vi "ServoController_check.vi"(7 "Servo Position Old (U16)":u16[][](array[numeric]), 8 "Error In":errorcluster, 11 "Servo Position In (U16)":u16[][](array[numeric])) -> (0 "Error Out":errorcluster, 3 "Servo Position Out (U16)":u16[][](array[numeric]))   [LabVIEW 2013]
uses:
  My Computer/Controls/Fin Status.ctl
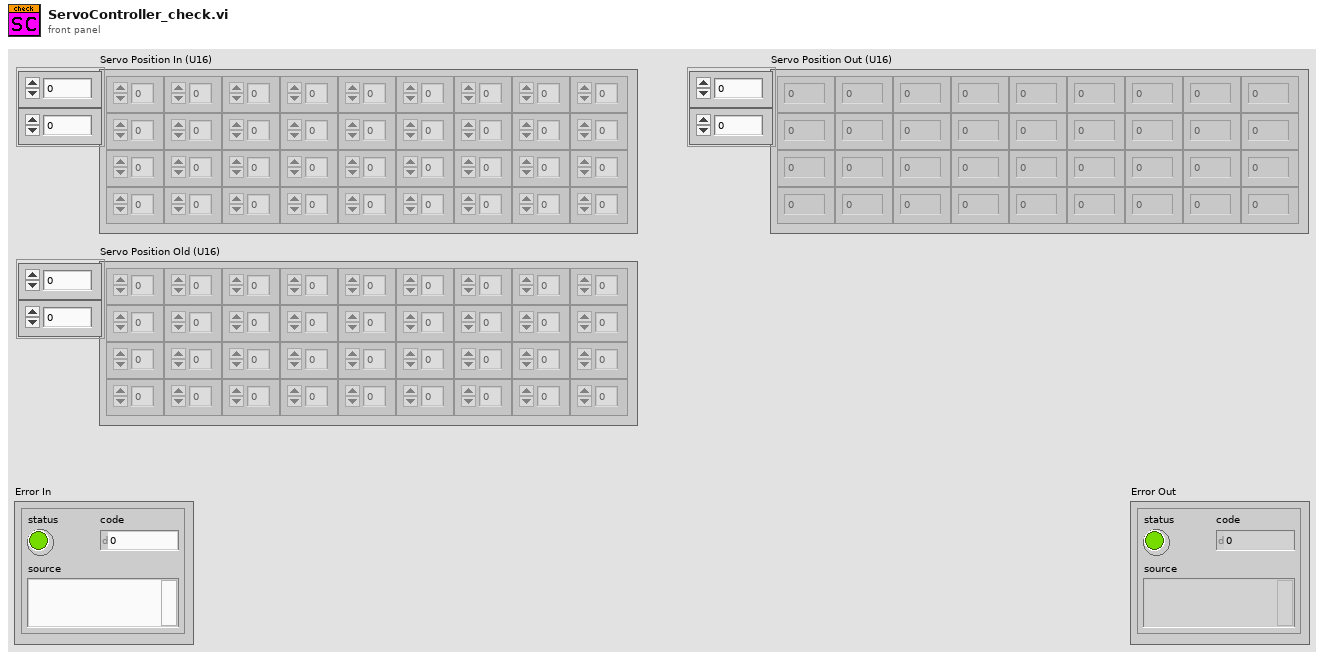
[diagram p1: front panel]
types:
  T1 = typedef "Fin Status.ctl" = u32[]
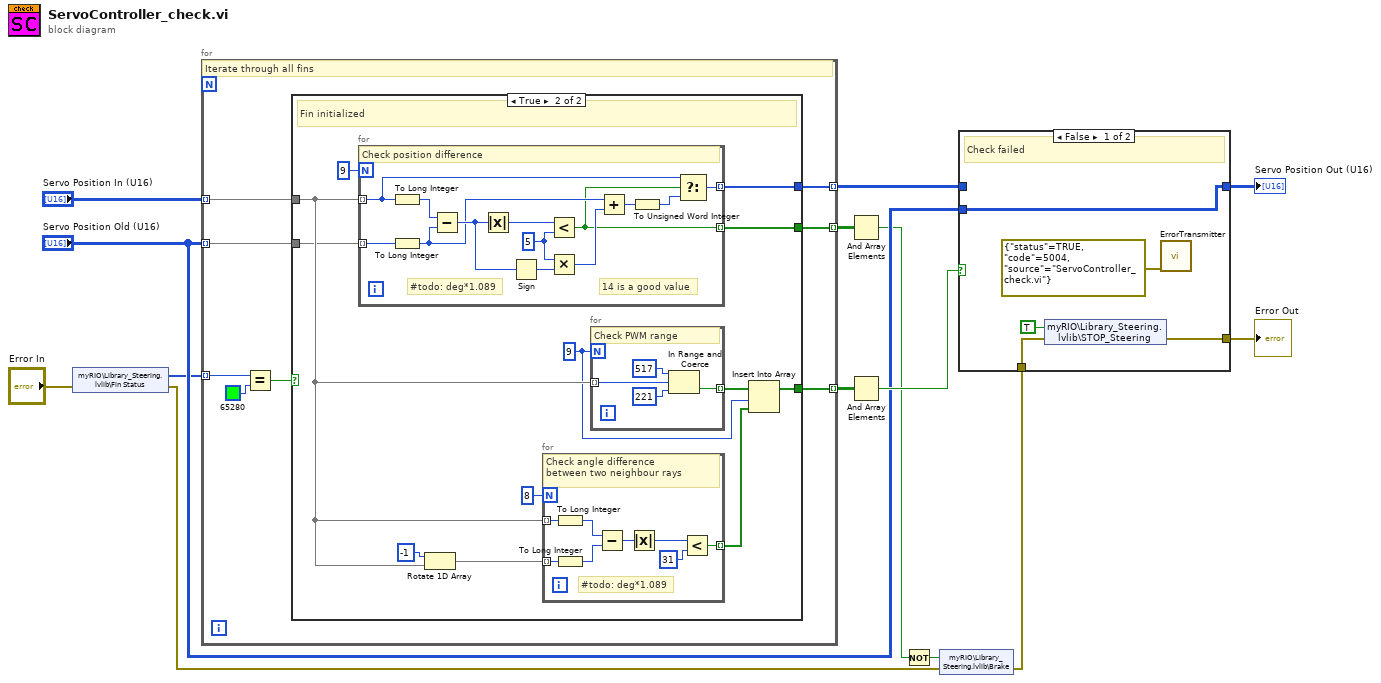
[diagram p0: block diagram]
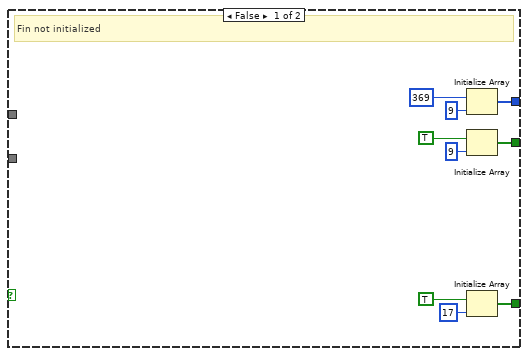
[diagram p3: hidden frame]
diagram:
  n1 = shared-variable "myRIO\\Library_Steering.lvlib\\Fin Status"(error in="Error In") -> (w8:T1, error out=w4:errorcluster)
  n2 = for {
    tunnel: [w22] -> w10 mode=indexing
    tunnel: "Servo Position In (U16)" -> [w21] mode=indexing
    tunnel: "Servo Position Old (U16)" -> [w20] mode=indexing
    tunnel: w8 -> [w19] mode=indexing
    tunnel: [w16] -> w13 mode=indexing
    tunnel: [w15] -> w6 mode=indexing
    # "Iterate through all fins"
    n3 = Equal?(x=w19, y=u32 65280 ("Round Color Box")) -> (x = y?=w17:bool)
    n4 = case shown="True" w17 {
      tunnel: [w26 w39] -> w22
      tunnel: w21 -> [_ w38]
      tunnel: w20 -> [_ w37]
      tunnel: [w27 w33] -> w16
      tunnel: [w23 w32] -> w15
      frame False {
        # "Fin not initialized"
        n5 = Initialize Array(u16 369 ("Numeric Indicator"), 9 ("dimension size")) -> (w26:u16[])
        n6 = Initialize Array(TRUE, 9 ("dimension size")) -> (w23:bool[])
        n7 = Initialize Array(TRUE, 17 ("dimension size")) -> (w27:bool[])
      }
      frame True {
        w34 = 9
        # "Fin initialized"
        n8 = for {
          N: 9 -> [_]
          tunnel: w38 -> [w54] mode=indexing
          tunnel: w37 -> [w56] mode=indexing
          tunnel: [w46] -> w39 mode=indexing
          tunnel: [w44] -> w32 mode=indexing
          w51 = 5 ("y")
          # "14 is a good value"
          # "#todo: deg*1.089"
          # "Check position difference"
          n9 = To Long Integer(number=w54) -> (32bit integer=w50:i32)
          n10 = To Long Integer(number=w56) -> (32bit integer=w45:i32)
          n11 = Subtract(x=w50, y=w45) -> (x-y=w53:i32)
          n12 = Absolute Value(x=w53) -> (abs(x)=w55:i32)
          n13 = Sign(1:w53) -> (0:w52:i32)
          n14 = Less?(x=w55, y=w51) -> (x < y?=w44:bool)
          n15 = Multiply(x=w51, y=w52) -> (x*y=w49:i32)
          n16 = Add(x=w45, y=w49) -> (x+y=w47:i32)
          n17 = To Unsigned Word Integer(number=w47) -> (unsigned 16bit integer=w48:u16)
          n18 = Select(t=w54, s=w44, f=w48) -> (s? t:f=w46:u16)
        }
        n19 = Rotate 1D Array(1:w38, 2:-1 ("n")) -> (0:w41:u16[])
        n20 = for {
          N: 8 -> [_]
          tunnel: w38 -> [w64] mode=indexing
          tunnel: w41 -> [w62] mode=indexing
          tunnel: [w57] -> w35 mode=indexing
          # "#todo: deg*1.089"
          # "Check angle difference\nbetween two neighbour rays"
          n21 = To Long Integer(number=w64) -> (32bit integer=w63:i32)
          n22 = To Long Integer(number=w62) -> (32bit integer=w61:i32)
          n23 = Subtract(x=w63, y=w61) -> (x-y=w60:i32)
          n24 = Absolute Value(x=w60) -> (abs(x)=w59:i32)
          n25 = Less?(x=w59, y=31) -> (x < y?=w57:bool)
        }
        n26 = for {
          N: w34 -> [_]
          tunnel: w38 -> [w65] mode=indexing
          tunnel: [w68] -> w36 mode=indexing
          # "Check PWM range"
          n27 = In Range and Coerce(upper limit=u16 517 ("y"), x=w65, lower limit=u16 221 ("y")) -> (In Range?=w68:bool)  [unwired: 1 out]
        }
        n28 = Insert Into Array(array=w36, index=w34, new element=w35) -> (w33:bool[])
      }
    }
  }
  n29 = And Array Elements(Boolean array=w6) -> (logical AND=w5:bool)
  n30 = And Array Elements(Boolean array=w13) -> (logical AND=w12:bool)
  n31 = Not(x=w5) -> (.not. x?=w1:bool)
  n32 = shared-variable "myRIO\\Library_Steering.lvlib\\Brake"(w1, error in=w4) -> (error out=w3:errorcluster)
  n33 = case shown="False" w12 {
    tunnel: [w73 w75] -> w11
    tunnel: w10 -> [_ w75]
    tunnel: "Servo Position Old (U16)" -> [w73 _]
    tunnel: w3 -> [w70 w74]
    tunnel: [w69 w74] -> w2
    frame False {
      # "Check failed"
      n34 = shared-variable "myRIO\\Library_Steering.lvlib\\STOP_Steering"(TRUE ("STOP_Steering"), error in=w70) -> (error out=w69:errorcluster)
      n35 = call "ErrorTransmitter.vi"("Error In"=errorcluster {"status"=TRUE, "code"=5004, "source"="ServoController_check.vi"} ("error constant")) -> ()  [unwired: 10 in, 1 out]
    }
    frame True {
      # "Check succeeded"
    }
  }
  "Error Out" <- w2
  "Servo Position Out (U16)" <- w11
